vi "Update Terminal Type from Child.vi"(8 "error in (no error)":errorcluster, 10 "Terminal Type":T1, 11 "Value Editor Base in":refnum<class "Value Editor Base.lvclass">) -> (0 "error out":errorcluster, 3 "Value Editor Base out":refnum<class "Value Editor Base.lvclass">)   [LabVIEW 2020, in "Value Editor Base.lvclass"]
uses:
  Value Editor Base.lvclass
  Value Editor Base.lvclass/Value Editor Base.ctl
  Terminal Mode.ctl
  FlexBlocks.lvlib
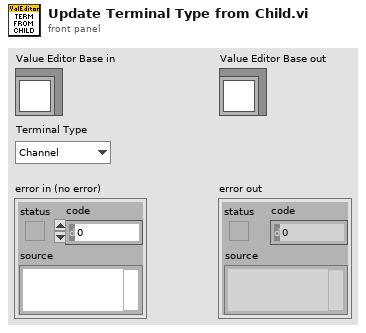
[diagram p1: front panel]
types:
  T1 = typedef "FlexBlocks.lvlib/Terminal Mode.ctl" = enum16{"Channel", "Config", "Value", "Control Ref"}
  T2 = typedef "Value Editor Base.lvclass/Ref Data.ctl" = cluster{"Type Descriptor":T3, "Terminal Mode":T1, "Value":variant}
  T3 = typedef "FlexBlocks.lvlib/Type Descriptor.ctl" = cluster{"Name":string, "Direction":T4, "Default":variant, "Min":variant, "Max":variant, "Step":variant, "Value Mode":T5, "Required":bool, "Connpane Index":i32, "Special Terminal":T6, "Color":u32, "Options":string[], "Type String":string, "Sort":i32, "Item Path":path}
  T4 = typedef "FlexBlocks.lvlib/Terminal Direction.ctl" = enum16{"Sink", "Source"}
  T5 = typedef "FlexBlocks.lvlib/Value Mode.ctl" = enum16{"Normal", "Range", "Select"}
  T6 = typedef "FlexBlocks.lvlib/Special Terminal.ctl" = enum16{"None", "Action", "Init", "Tag", "State in", "State out", "Error"}
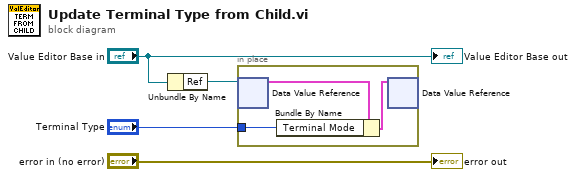
[diagram p0: block diagram]
diagram:
  n1 = Unbundle By Name("Value Editor Base in") -> ("Ref"=w3:refnum<data-value>)
  n2 = in-place {
    in-place-border: "Terminal Type" -> [w5]
    n3 = in-place-dvr #1(w3) -> (w7:T2)  [unwired: 1 out]
    n4 = Bundle By Name(cluster=w7, "Terminal Mode"=w5) -> (w6:T2)
    n5 = in-place-dvr #1(w6) -> ()  [unwired: 2 out]
  }
  "error out" <- "error in (no error)"
  "Value Editor Base out" <- "Value Editor Base in"
